vi "总磷通讯.vi"() -> ()   [LabVIEW 2016, in "斯坦道总磷.lvlib"]
uses:
  <vilib>/NI/Modbus Library/API/Wrapper/Create TCP Slave.vi
  <vilib>/Utility/config.llb/Write Key (Boolean).vi
  <vilib>/Utility/config.llb/Write Key (String).vi
  <vilib>/Plasmionique/MB Master/MB_Master/MB_Master.lvclass
  <vilib>/NI/Modbus Library/API/slave/Modbus Slave.lvclass
  <vilib>/Utility/config.llb/NI_LVConfig.lvlib
  <vilib>/Plasmionique/MB Master/MB Master.lvlib
  <vilib>/NI/Modbus Library/API/Wrapper/API Main.lvlib
panel:
  out "总氮测量数据区":u16[](array[numeric])
  out "总氮状态告警区":u16[](array[numeric])
  out "总磷状态告警区":u16[](array[numeric])
  out "总磷测量数据区":u16[](array[numeric])
  out "序列号":string
  out "状态告警区":T1
  out "测量数据区":T2 {"单位" items=["ug/L", "mg/L", "ppm", "mg/m3", "cm", "ppb", "ug/m3", "%", "nmol/mol", "umol/mol", "MPN/L", "MPN/100ml", "ng/m3", "NTU", "无量纲", "ms/cm", "us/cm", "℃", "mV", "万个/L"]}
  out "status":bool
  out "关键参数区":T3
  in  "读关键参数区":bool
  in  "读状态告警区":bool
  in  "读测量数据区":bool
  in  "站号":u16(ring) items=["总磷"=1, "氨氮"=3]
  in  "停止":bool
  in  "启动":bool
  in  "控制命令":u16(ring) items=["启动测量"=1, "标样核查"=2, "零点核查"=3, "跨度核查"=4, "空白测试"=5, "平行样测试"=6, "加标回收"=7, "空白校准"=8, "标样校准"=9, "初始化（清洗）"=10, "停止测试"=11, "仪器重启"=12, "校时"=13, "模式设置"=14, "测量间隔设置"=15]
  in  "控制命令参数":u16[](array[numeric]) format="%04xH"
  in  "VISA Resource":refnum<visa-resource-name>
  in  "启用模块":bool
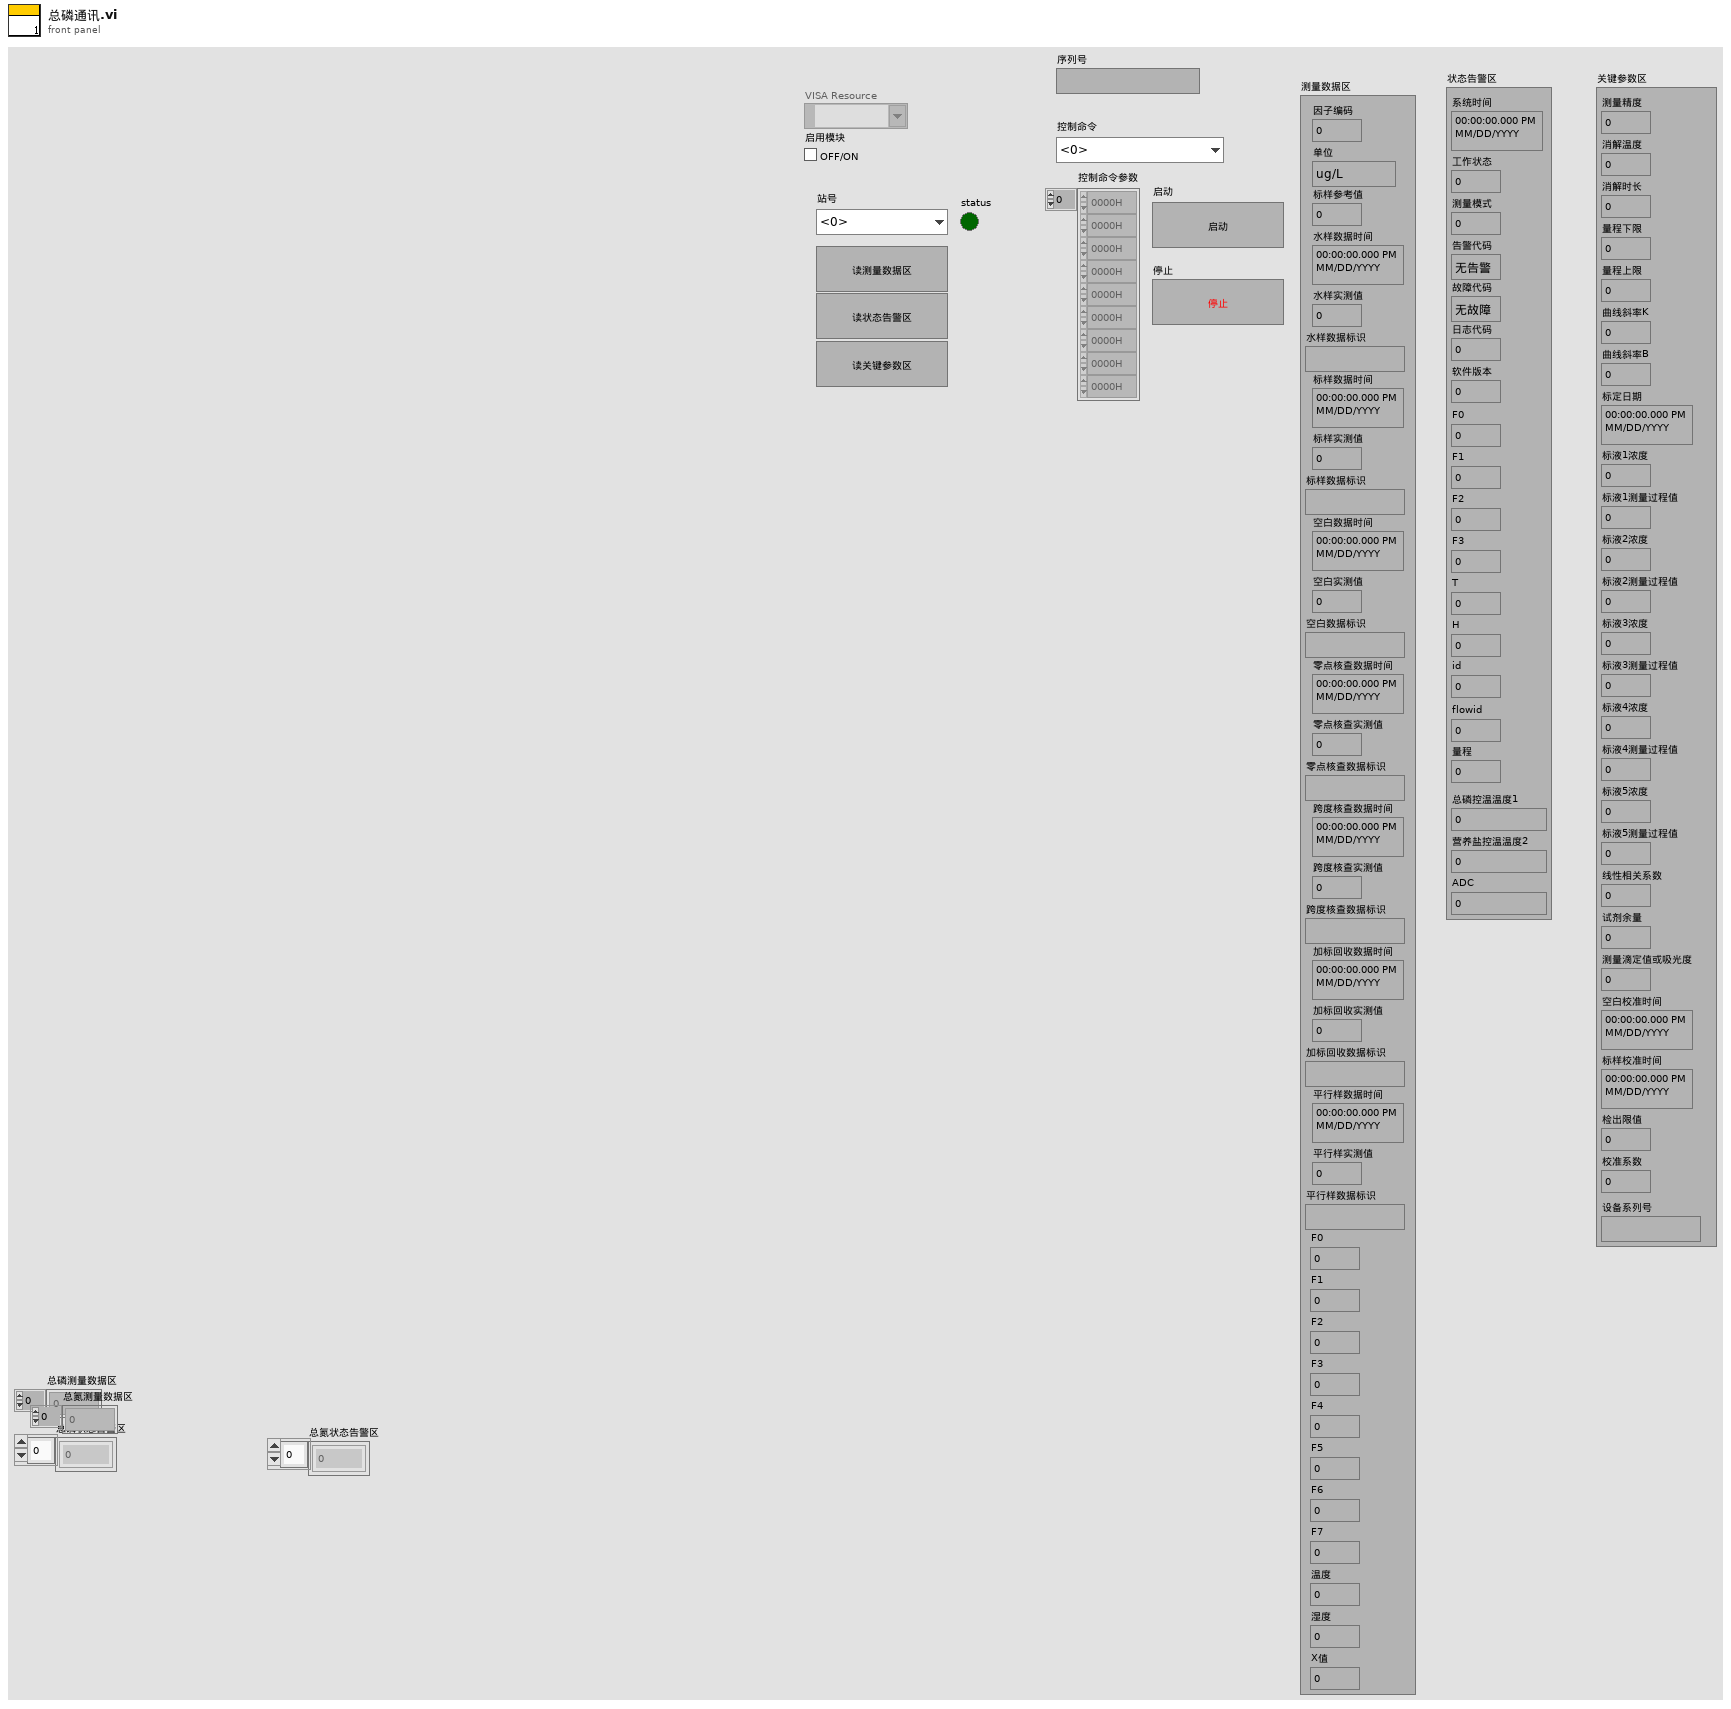
[diagram p1: front panel]
types:
  T1 = cluster{"系统时间":timestamp, "工作状态":u16, "测量模式":u16, "告警代码":enum16{"无告警", "缺试剂告警", "缺水样告警", "缺蒸馏水告警", "缺标液告警", "仪表漏液告警", "标定异常告警", "超量程告警", "加热异常", "低试剂预警", "超上限告警", "超下限告警", "仪表内部其他异常", "滴定异常告警", "电极异常告警", "量程切换告警", "参数设置告警", "PH电极电位异常", "电导率电极异常", "浊度光度异常", "溶解氧电极异常", "溶解氧光强异常", "温度异常告警", "PH异常告警", "溶解氧异常告警", "电导率异常告警", "浊度异常告警", "叶绿素异常告警", "藻密度异常告警", "蓝绿藻异常告警", "ORP异常告警", "氨氮异常告警", "清洁刷异常告警", "SD卡异常告警", "蓝牙异常告警", "Wifi异常告警", "流程异常告警"}, "故障代码":enum16{"无故障", "电机故障", "温度故障", "通讯故障", "滴定故障"}, "日志代码":u16, "软件版本":u16, "F0":sgl, "F1":sgl, "F2":sgl, "F3":sgl, "T":sgl, "H":sgl, "id":u16, "flowid":u16, "量程":u16, "总磷控温温度1":sgl, "营养盐控温温度2":sgl, "ADC":sgl}
  T2 = cluster{"因子编码":u32, "单位":u16, "标样参考值":sgl, "水样数据时间":timestamp, "水样实测值":sgl, "水样数据标识":string, "标样数据时间":timestamp, "标样实测值":sgl, "标样数据标识":string, "空白数据时间":timestamp, "空白实测值":sgl, "空白数据标识":string, "零点核查数据时间":timestamp, "零点核查实测值":sgl, "零点核查数据标识":string, "跨度核查数据时间":timestamp, "跨度核查实测值":sgl, "跨度核查数据标识":string, "加标回收数据时间":timestamp, "加标回收实测值":sgl, "加标回收数据标识":string, "平行样数据时间":timestamp, "平行样实测值":sgl, "平行样数据标识":string, "F0":sgl, "F1":sgl, "F2":sgl, "F3":sgl, "F4":sgl, "F5":sgl, "F6":sgl, "F7":sgl, "温度":sgl, "湿度":sgl, "X值":sgl}
  T3 = cluster{"测量精度":u16, "消解温度":u16, "消解时长":u16, "量程下限":sgl, "量程上限":sgl, "曲线斜率K":sgl, "曲线斜率B":sgl, "标定日期":timestamp, "标液1浓度":sgl, "标液1测量过程值":sgl, "标液2浓度":sgl, "标液2测量过程值":sgl, "标液3浓度":sgl, "标液3测量过程值":sgl, "标液4浓度":sgl, "标液4测量过程值":sgl, "标液5浓度":sgl, "标液5测量过程值":sgl, "线性相关系数":sgl, "试剂余量":u32, "测量滴定值或吸光度":sgl, "空白校准时间":timestamp, "标样校准时间":timestamp, "检出限值":sgl, "校准系数":sgl, "设备系列号":string}
  T4 = typedef "NI_LVConfig.lvlib/Config Data RefNum.ctl" = refnum<k1>
  T5 = enum8{"Enabled", "Disabled", "Disabled and Grayed Out"}
  T6 = cluster{"系统时间":timestamp, "工作状态":enum16{"空闲", "水样测试", "标样核查", "零点核查", "跨度核查", "空白测试", "平行样测试", "加标回收", "空白校准", "标样校准", "初始化（清洗）"}, "测量模式":enum16{"待机", "连续模式", "周期模式", "定点模式", "受控模式", "手动模式"}, "告警代码":enum16{"无告警", "缺试剂告警", "缺水样告警", "缺蒸馏水告警", "缺标液告警", "仪表漏液告警", "标定异常告警", "超量程告警", "加热异常", "低试剂预警", "超上限告警", "超下限告警", "仪表内部其他异常", "滴定异常告警", "电极异常告警", "量程切换告警", "参数设置告警", "PH电极电位异常", "电导率电极异常", "浊度光度异常", "溶解氧电极异常", "溶解氧光强异常", "温度异常告警", "PH异常告警", "溶解氧异常告警", "电导率异常告警", "浊度异常告警", "叶绿素异常告警", "藻密度异常告警", "蓝绿藻异常告警", "ORP异常告警", "氨氮异常告警", "清洁刷异常告警", "SD卡异常告警", "蓝牙异常告警", "Wifi异常告警", "流程异常告警"}, "故障代码":enum16{"无故障", "电机故障", "温度故障", "通讯故障", "滴定故障"}, "日志代码":u16, "软件版本":u16, "F0":sgl, "F1":sgl, "F2":sgl, "F3":sgl, "T":sgl, "H":sgl, "id":u16, "flowid":u16, "量程":u16, "总磷控温温度1":sgl, "营养盐控温温度2":sgl, "ADC":sgl}
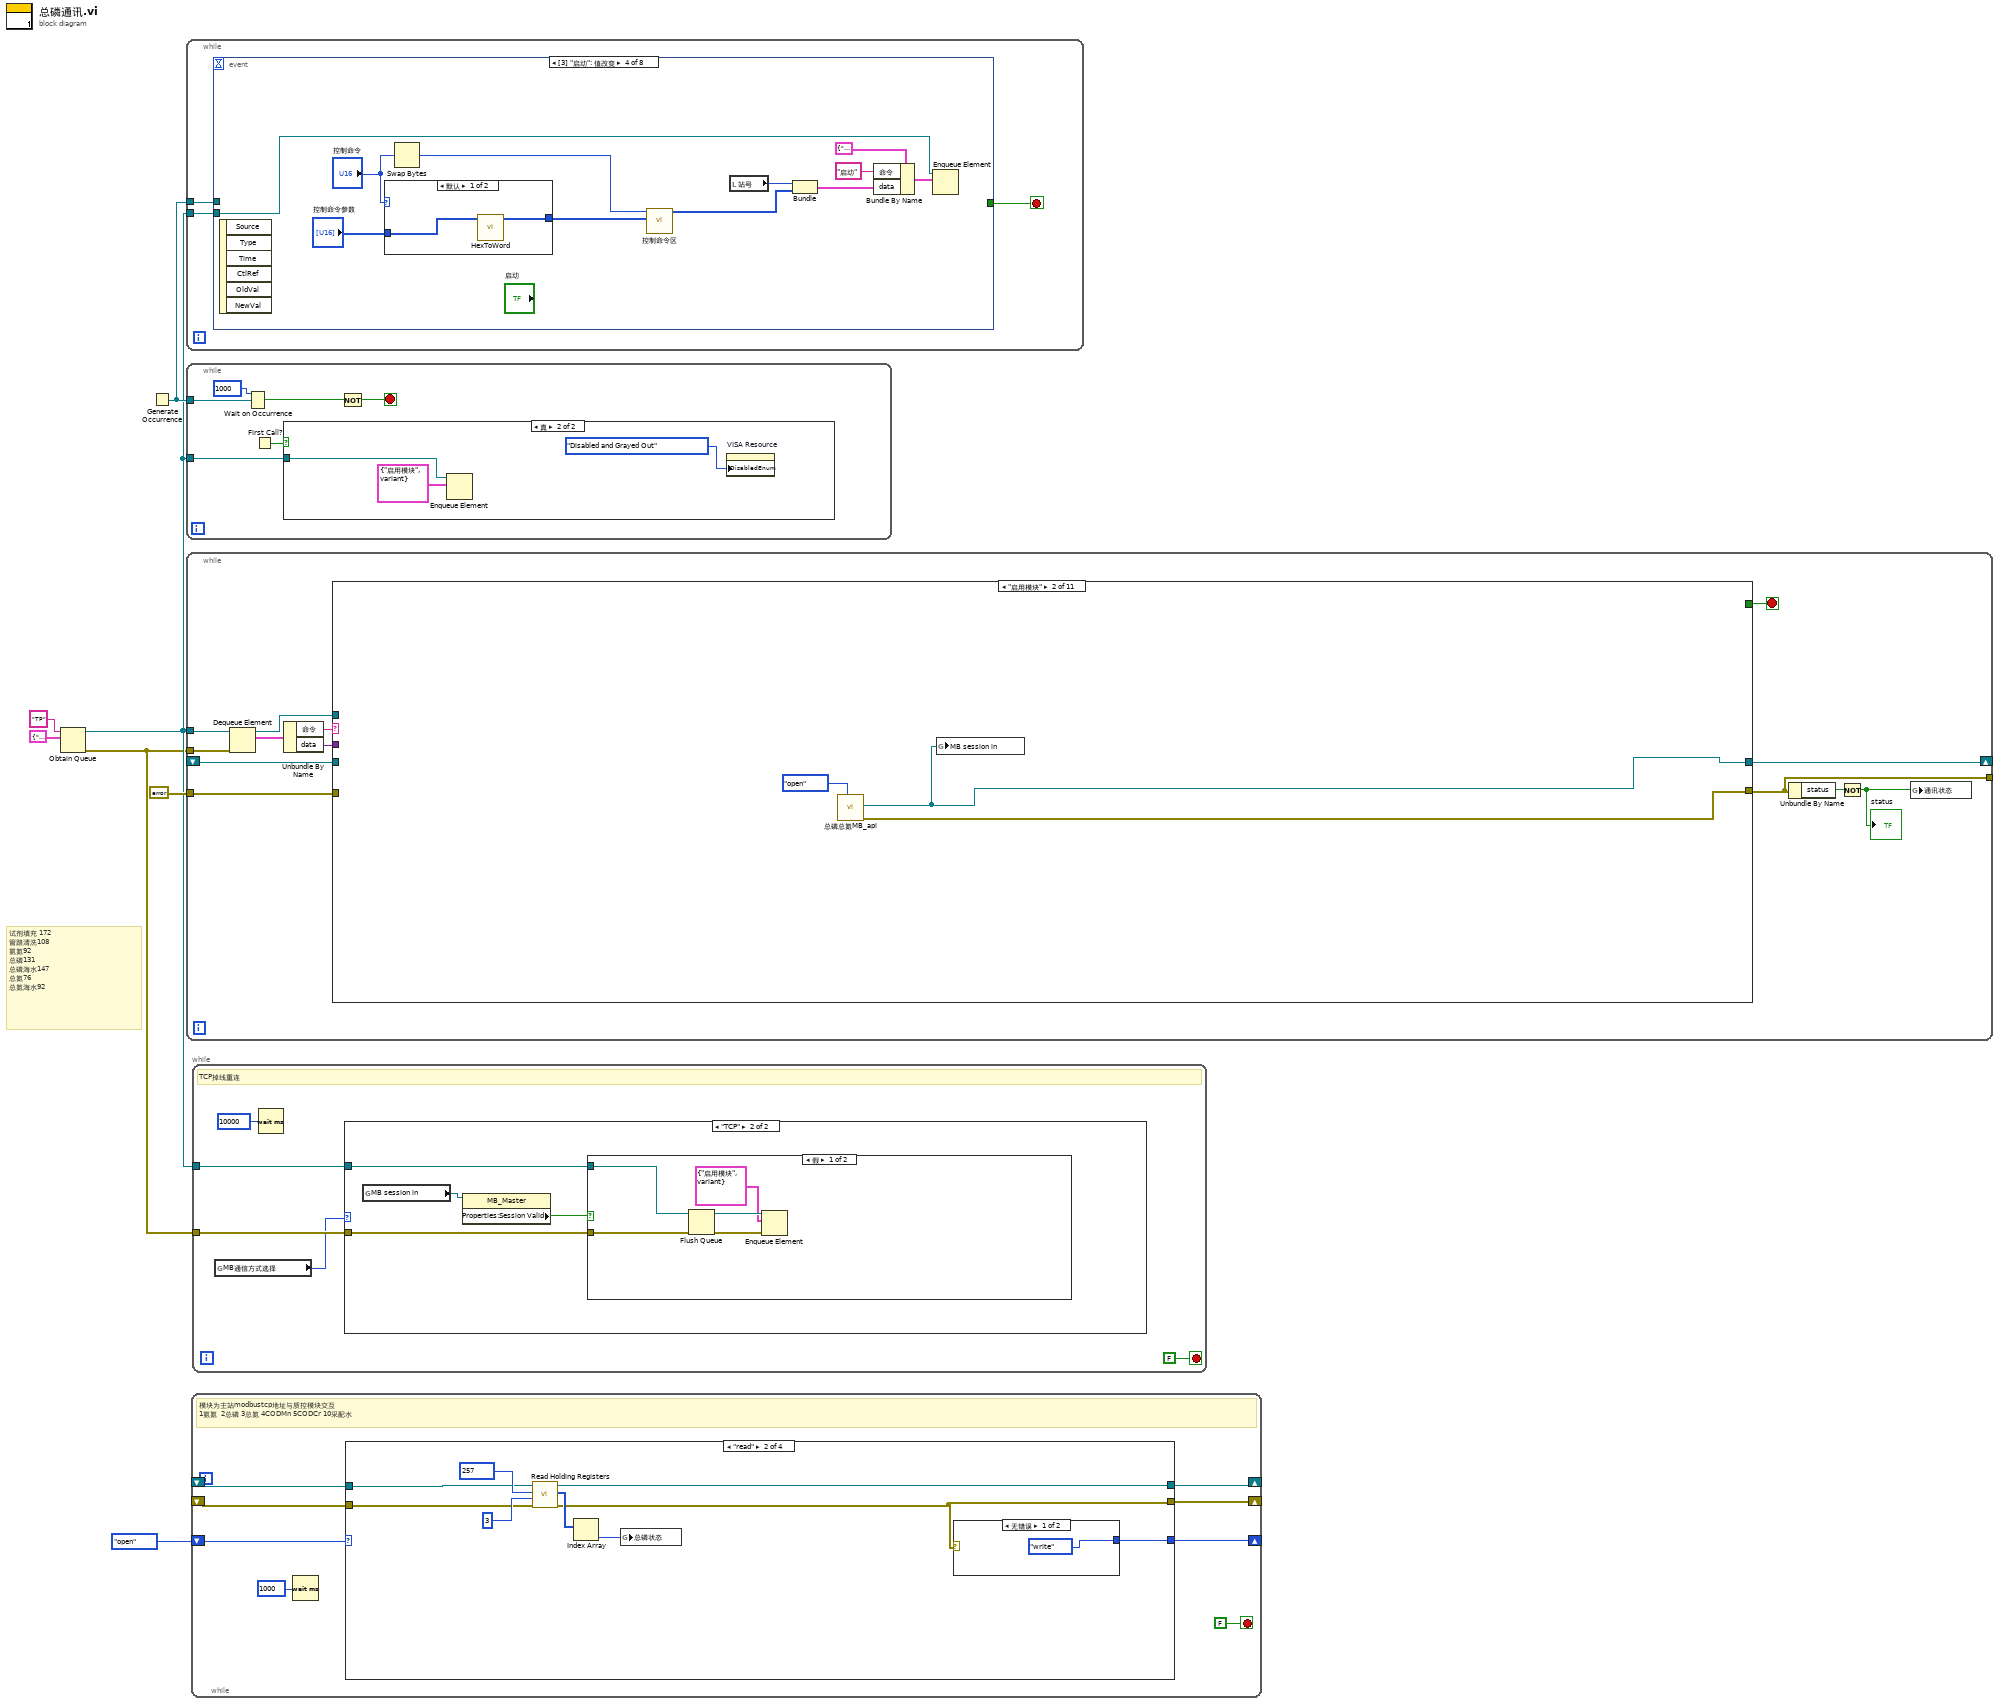
[diagram p0: block diagram]
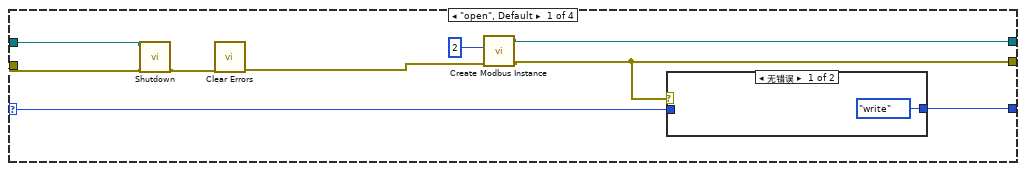
[diagram p4: hidden frame]
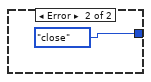
[diagram p6: hidden frame]
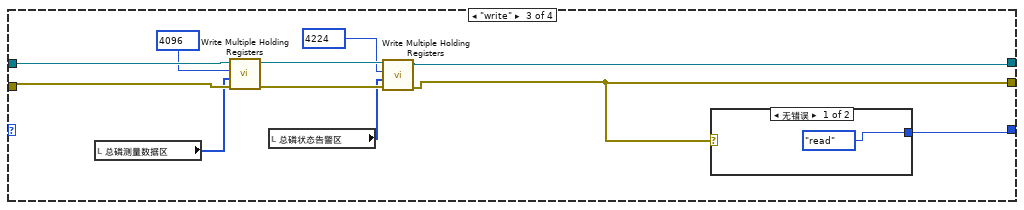
[diagram p7: hidden frame]
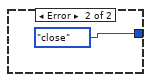
[diagram p8: hidden frame]
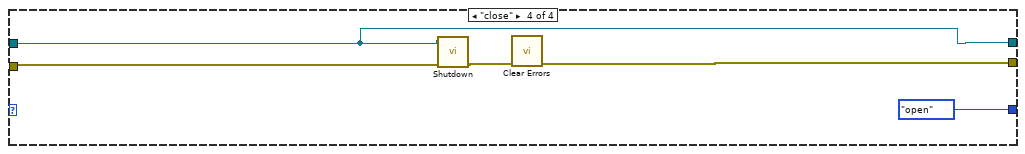
[diagram p9: hidden frame]
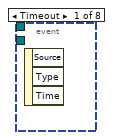
[diagram p11: hidden frame]
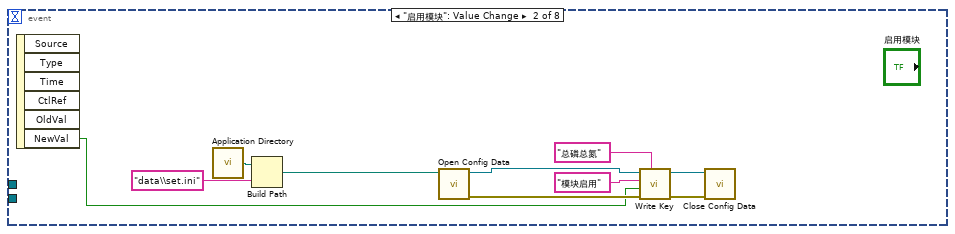
[diagram p12: hidden frame]
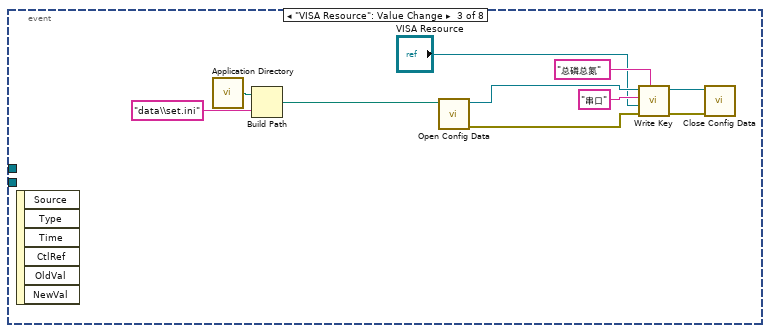
[diagram p13: hidden frame]
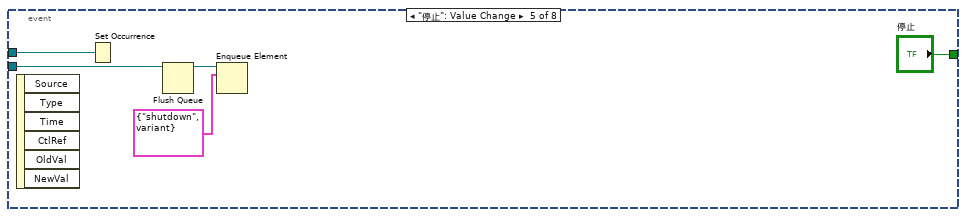
[diagram p15: hidden frame]
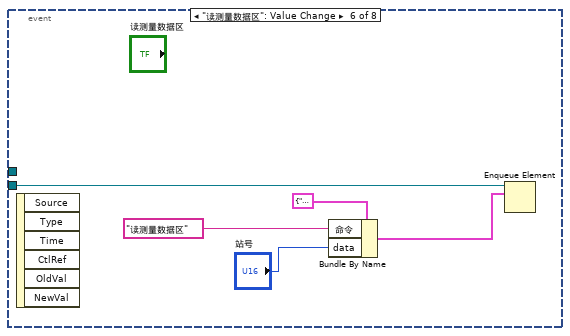
[diagram p16: hidden frame]
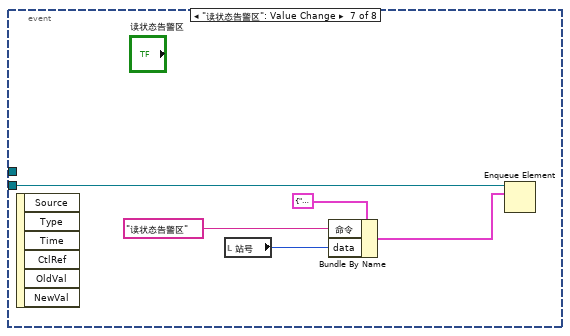
[diagram p17: hidden frame]
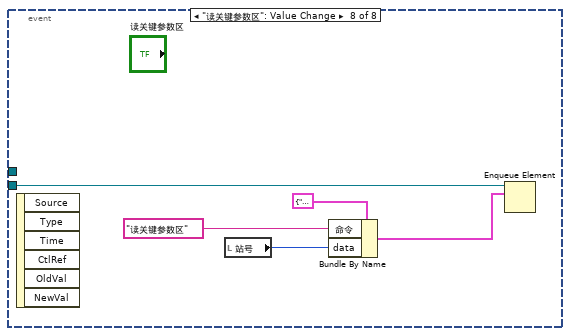
[diagram p18: hidden frame]
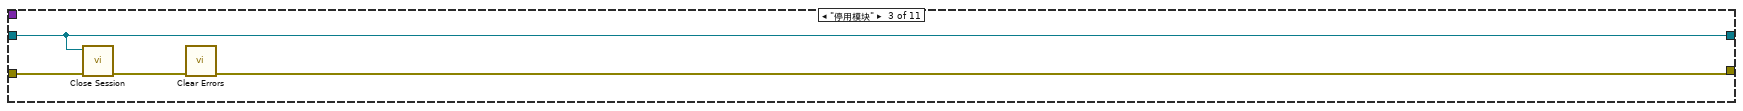
[diagram p20: hidden frame]
diagram:
  # "试剂填充 172 \n管路清洗108\n氨氮92\n总磷131\n总磷海水147\n总氮76\n总氮海水92"
  n1 = Obtain Queue(name (unnamed)="TP" ("名称（未命名）"), element data type=cluster{"命令":string, "data":variant} {"命令"="", "data"=variant}) -> (queue out=w2:refnum<queue>, error out=w1:errorcluster)  [unwired: 3 in, 1 out]
  n2 = Generate Occurrence() -> (w4:refnum<k4>)
  n3 = while {
    tunnel: w2 -> [w10]
    tunnel: w4 -> [w8]
    stop <- w9 stop-if-true
    n4 = event shown="[3] \"启动\": 值改变" {
      selector: _ -> [_ _ _ _ _ _ _ _]
      dyn-events: _ -> [_ _ _ _ _ _ _ _]
      timeout: _ -> [_ _ _ _ _ _ _ _]
      tunnel: w10 -> [_ _ _ w41 w48 w54 w59 w64]
      tunnel: [_ _ _ _ "停止" _ _ _] -> w9
      tunnel: w8 -> [_ _ _ _ w45 _ _ _]
      event Timeout {
        n5 = event-data() -> ()  [unwired: 1 in, 3 out]
      }
      event "启用模块": Value Change {
        n6 = event-data() -> ("NewVal"=w11:bool)  [unwired: 1 in, 5 out]
        n7 = call <vilib>:"Application Directory.vi"() -> ("Application Directory"=w13:path)
        n8 = Build Path(base path=w13, name or relative path="data\\set.ini" ("名称或相对路径")) -> (appended path=w14:path)
        n9 = call <vilib>:"Open Config Data.vi"("configuration file path"=w14) -> ("error out"=w20:errorcluster, "refnum"=w19:T4)  [unwired: 8 in, 1 out]
        n10 = call-poly <vilib>:"Write Key.vi"("section"="总磷总氮", "error in (no error)"=w20, "value"=w11, "key"="模块启用", "refnum"=w19) -> ("error out"=w16:errorcluster, "refnum out"=w12:T4)  [unwired: 4 in, 1 out]
        n11 = call <vilib>:"Close Config Data.vi"("error in (no error)"=w16, "refnum"=w12) -> ()  [unwired: 8 in, 2 out]
      }
      event "VISA Resource": Value Change {
        n12 = event-data() -> ()  [unwired: 1 in, 6 out]
        n13 = call <vilib>:"Application Directory.vi"() -> ("Application Directory"=w23:path)
        n14 = Build Path(base path=w23, name or relative path="data\\set.ini" ("名称或相对路径")) -> (appended path=w24:path)
        n15 = call <vilib>:"Open Config Data.vi"("configuration file path"=w24) -> ("error out"=w30:errorcluster, "refnum"=w29:T4)  [unwired: 8 in, 1 out]
        n16 = call-poly <vilib>:"Write Key.vi"("section"="总磷总氮", "error in (no error)"=w30, "value"="VISA Resource", "key"="串口", "refnum"=w29) -> ("error out"=w26:errorcluster, "refnum out"=w22:T4)  [unwired: 4 in, 1 out]
        n17 = call <vilib>:"Close Config Data.vi"("error in (no error)"=w26, "refnum"=w22) -> ()  [unwired: 8 in, 2 out]
      }
      event "启动": Value Change {
        n18 = event-data() -> ()  [unwired: 1 in, 6 out]
        n19 = case shown="默认" "控制命令" {
          tunnel: "控制命令参数" -> [w43 w44]
          tunnel: [w42 w44] -> w31
          frame Default {
            n20 = call "HexToWord.vi"("数组"=w43) -> ("WORD"=w42:u16[])  [unwired: 10 in]
          }
          frame 13 {
          }
        }
        n21 = Swap Bytes(anything="控制命令") -> (byte swapped=w34:u16)
        n22 = call "控制命令区.vi"("控制命令参数"=w31, "控制命令"=w34) -> ("控制命令"=w37:u16[])  [unwired: 9 in]
        n23 = local read "站号"() -> (w36:u16)
        n24 = Bundle("站号"=w36, "控制命令"=w37) -> (w35:cluster{"站号":u16, "控制命令":u16[]})  [unwired: 1 in]
        n25 = Bundle By Name(cluster=cluster{"命令":string, "data":variant} {"命令"="", "data"=variant} ("元素"), "命令"="启动", "data"=w35) -> (w39:cluster{"命令":string, "data":variant})
        n26 = Enqueue Element(queue=w41, element=w39) -> ()  [unwired: 2 in, 3 out]
      }
      event "停止": Value Change {
        n27 = event-data() -> ()  [unwired: 1 in, 6 out]
        n28 = Set Occurrence(w45) -> ()
        n29 = Flush Queue(queue=w48) -> (queue out=w47:refnum<queue>)  [unwired: 1 in, 2 out]
        n30 = Enqueue Element(queue=w47, element=cluster{"命令":string, "data":variant} {"命令"="shutdown", "data"=variant} ("元素")) -> ()  [unwired: 2 in, 3 out]
      }
      event "读测量数据区": Value Change {
        n31 = event-data() -> ()  [unwired: 1 in, 6 out]
        n32 = Bundle By Name(cluster=cluster{"命令":string, "data":variant} {"命令"="", "data"=variant} ("元素"), "命令"="读测量数据区", "data"="站号") -> (w52:cluster{"命令":string, "data":variant})
        n33 = Enqueue Element(queue=w54, element=w52) -> ()  [unwired: 2 in, 3 out]
      }
      event "读状态告警区": Value Change {
        n34 = event-data() -> ()  [unwired: 1 in, 6 out]
        n35 = local read "站号"() -> (w55:u16)
        n36 = Bundle By Name(cluster=cluster{"命令":string, "data":variant} {"命令"="", "data"=variant} ("元素"), "命令"="读状态告警区", "data"=w55) -> (w57:cluster{"命令":string, "data":variant})
        n37 = Enqueue Element(queue=w59, element=w57) -> ()  [unwired: 2 in, 3 out]
      }
      event "读关键参数区": Value Change {
        n38 = event-data() -> ()  [unwired: 1 in, 6 out]
        n39 = local read "站号"() -> (w60:u16)
        n40 = Bundle By Name(cluster=cluster{"命令":string, "data":variant} {"命令"="", "data"=variant} ("元素"), "命令"="读关键参数区", "data"=w60) -> (w62:cluster{"命令":string, "data":variant})
        n41 = Enqueue Element(queue=w64, element=w62) -> ()  [unwired: 2 in, 3 out]
      }
    }
  }
  n42 = while {
    tunnel: w4 -> [w70]
    tunnel: w2 -> [w66]
    stop <- w67 stop-if-true
    n43 = Wait on Occurrence(2:w70, 3:1000 ("毫秒超时(-1)")) -> (0:w68:bool)  [unwired: 1 in]
    n44 = First Call?() -> (First Call?: T/F=w65:bool)
    n45 = case shown="真" w65 {
      tunnel: w66 -> [_ w72]
      frame False {
      }
      frame True {
        n46 = Enqueue Element(queue=w72, element=cluster{"命令":string, "data":variant} {"命令"="启用模块", "data"=variant} ("元素")) -> ()  [unwired: 2 in, 3 out]
        n47 = property on="VISA Resource" class="VISAName"("DisabledEnum"=T5."Disabled and Grayed Out" ("禁用")) -> ()  [unwired: 2 in, 2 out]
      }
    }
    n48 = Not(x=w68) -> (.not. x?=w67:bool)
  }
  n49 = while {
    tunnel: w2 -> [w86]
    tunnel: w1 -> [w85]
    shift-right: [w83] -> _
    shift-left: _ -> [w82]
    tunnel: errorcluster {"status"=FALSE, "code"=0, "source"=""} ("error out") -> [w81]
    tunnel: [w76] -> _
    stop <- w84 stop-if-true
    n50 = Dequeue Element(queue=w86, error in (no error)=w85) -> (queue out=w77:refnum<queue>, element=w79:cluster{"命令":string, "data":variant})  [unwired: 1 in, 2 out]
    n51 = Unbundle By Name(w79) -> ("命令"=w80:string, "data"=w78:variant)
    n52 = case shown="\"启用模块\"" w80 {
      tunnel: w78 -> [_ _ _ w105 w116 w133 w143 w157 w175 w189 _]
      tunnel: w77 -> [_ _ _ _ _ _ _ _ _ _ w202]
      tunnel: [_ _ _ _ _ _ _ _ _ _ TRUE] -> w84
      tunnel: [w87 w90 w92 w108 w119 w135 w147 w166 w182 w196 w198] -> w83
      tunnel: [w88 w89 w93 w107 w118 w134 w148 w156 w183 w197 w199] -> w76
      tunnel: w82 -> [w87 _ w92 w104 w115 w132 w142 w160 w178 w192 w198]
      tunnel: w81 -> [w88 _ w95 w101 w112 w129 w140 w161 w179 w193 w200]
      frame Default {
      }
      frame "启用模块" {
        n53 = call "总磷总氮MB_api.vi"("STEP"=enum16{"open", "read", "write", "close"}."open") -> ("error out"=w89:errorcluster, "MB session out"=w90:refnum<class "MB_Master.lvclass">)  [unwired: 8 in, 1 out]
        n54 = global write "VAR总磷全局变量.vi" "MB session in"(w90) -> ()
      }
      frame "停用模块" {
        n55 = call-dynamic "Close Session.vi"("error in (no error)"=w95, "MB session in"=w92) -> ("error out"=w94:errorcluster)  [unwired: 9 in]
        n56 = call <vilib>:"Clear Errors.vi"("error in (no error)"=w94) -> ("error out"=w93:errorcluster)  [unwired: 5 in, 1 out]
      }
      frame "启动" {
        n57 = Variant To Data(type=cluster{"站号":u16, "控制命令":u16[]} {"站号"=0, "控制命令"=[]} ("输出簇"), Variant=w105) -> (data=w99:cluster{"站号":u16, "控制命令":u16[]})  [unwired: 1 in, 1 out]
        n58 = Unbundle By Name(w99) -> ("站号"=w98:u16, "控制命令"=w96:u16[])
        n59 = property class="MB_Master"(reference=w104, error in=w101, "Properties:Slave ID"=w98) -> (reference out=w103:refnum<class "MB_Master.lvclass">, error out=w102:errorcluster)
        n60 = Index Array(array=w96) -> (element=w97:u16)  [unwired: 1 in]
        n61 = global write "VAR总磷全局变量.vi" "控制命令"(w97) -> ()
        n62 = call <vilib>:"Write Multiple Registers.vi"("error in (no error)"=w102, "values"=w96, "starting address"=u16 4608, "MB session in"=w103) -> ("error out"=w107:errorcluster, "MB session out"=w108:refnum<class "MB_Master.lvclass">)  [unwired: 6 in]
      }
      frame "盲样测试" {
        n63 = Variant To Data(type=0, Variant=w116) -> (data=w109:i32)  [unwired: 1 in, 1 out]
        n64 = case shown="默认" w109 {
          tunnel: [u16[] [] ("values") u16[] [33539, 0] ("values") u16[] [23555, 0] ("values")] -> w111
          frame Default {
          }
          frame 1 {
            # "总磷盲样测试命令"
          }
          frame 3 {
            # "氨氮盲样测试"
          }
        }
        n65 = property class="MB_Master"(reference=w115, error in=w112, "Properties:Slave ID"=w109) -> (reference out=w114:refnum<class "MB_Master.lvclass">, error out=w113:errorcluster)
        n66 = call <vilib>:"Write Multiple Registers.vi"("error in (no error)"=w113, "values"=w111, "starting address"=u16 24592, "MB session in"=w114) -> ("error out"=w118:errorcluster, "MB session out"=w119:refnum<class "MB_Master.lvclass">)  [unwired: 6 in]
      }
      frame "debug" {
        n67 = Variant To Data(type=cluster{"站号":u16, "控制命令":u16[]} {"站号"=0, "控制命令"=[]} ("输出簇"), Variant=w133) -> (data=w127:cluster{"站号":u16, "控制命令":u16[]})  [unwired: 1 in, 1 out]
        n68 = Unbundle By Name(w127) -> ("站号"=w126:u16, "控制命令"=w124:u16[])
        n69 = property class="MB_Master"(reference=w132, error in=w129, "Properties:Slave ID"=w126) -> (reference out=w131:refnum<class "MB_Master.lvclass">, error out=w130:errorcluster)
        n70 = Index Array(array=w124) -> (element=w125:u16)  [unwired: 1 in]
        n71 = global write "VAR总磷全局变量.vi" "控制命令"(w125) -> ()
        n72 = call <vilib>:"Write Multiple Registers.vi"("error in (no error)"=w130, "values"=w124, "starting address"=u16 24594, "MB session in"=w131) -> ("error out"=w134:errorcluster, "MB session out"=w135:refnum<class "MB_Master.lvclass">)  [unwired: 6 in]
      }
      frame "读测量数据区" {
        n73 = Variant To Data(type=u8 1 ("Slave ID"), Variant=w143) -> (data=w138:u8)  [unwired: 1 in, 1 out]
        n74 = property class="MB_Master"(reference=w142, error in=w140, "Properties:Slave ID"=w138) -> (reference out=w141:refnum<class "MB_Master.lvclass">, error out=w139:errorcluster)
        n75 = call <vilib>:"Read Holding Registers.vi"("error in (no error)"=w139, "quantity"=u16 104, "starting address"=u16 4096, "MB session in"=w141) -> ("error out"=w148:errorcluster, "Registers"=w137:u16[], "MB session out"=w147:refnum<class "MB_Master.lvclass">)  [unwired: 5 in]
        n76 = call "测量数据区.vi"("数组"=w137) -> ("测量数据区"=w136:T2)  [unwired: 10 in]
        "测量数据区" <- w136
        n77 = case shown="2" w138 {
          tunnel: w136 -> [_ w149 w151]
          tunnel: w137 -> [_ w150 w152]
          frame 0, Default {
          }
          frame 1 {
            n78 = global write "VAR总磷全局变量.vi" "总磷测量数据区"(w149) -> ()
            "总磷测量数据区" <- w150
          }
          frame 2 {
            n79 = global write "VAR总磷全局变量.vi" "总氮测量数据区"(w151) -> ()
            "总氮测量数据区" <- w152
          }
        }
        n80 = global write "VAR总磷全局变量.vi" "测量数据区"(w136) -> ()
      }
      frame "读状态告警区" {
        n81 = Variant To Data(type=u8 1 ("Slave ID"), Variant=w157) -> (data=w162:u8)  [unwired: 1 in, 1 out]
        n82 = property class="MB_Master"(reference=w160, error in=w161, "Properties:Slave ID"=w162) -> (reference out=w159:refnum<class "MB_Master.lvclass">, error out=w158:errorcluster)
        n83 = call <vilib>:"Read Holding Registers.vi"("error in (no error)"=w158, "quantity"=u16 29, "starting address"=u16 4224, "MB session in"=w159) -> ("error out"=w156:errorcluster, "Registers"=w153:u16[], "MB session out"=w166:refnum<class "MB_Master.lvclass">)  [unwired: 5 in]
        n84 = call "状态告警区.vi"("数组"=w153) -> ("状态告警区"=w154:T6)  [unwired: 10 in]
        "状态告警区" <- w154
        n85 = global write "VAR总磷全局变量.vi" "状态告警区"(w154) -> ()
        n86 = Unbundle By Name(w154) -> ("id"=w155:u16)
        n87 = case shown="2, 76" w155 {
          tunnel: w154 -> [_ w167 w169]
          tunnel: w153 -> [_ w168 w170]
          frame 0, Default {
          }
          frame 1, 131 {
            n88 = global write "VAR总磷全局变量.vi" "总磷状态告警区"(w167) -> ()
            "总磷状态告警区" <- w168
          }
          frame 2, 76 {
            n89 = global write "VAR总磷全局变量.vi" "总氮状态告警区"(w169) -> ()
            "总氮状态告警区" <- w170
          }
        }
      }
      frame "读关键参数区" {
        n90 = Variant To Data(type=u8 1 ("Slave ID"), Variant=w175) -> (data=w173:u8)  [unwired: 1 in, 1 out]
        n91 = property class="MB_Master"(reference=w178, error in=w179, "Properties:Slave ID"=w173) -> (reference out=w177:refnum<class "MB_Master.lvclass">, error out=w176:errorcluster)
        n92 = call <vilib>:"Read Holding Registers.vi"("error in (no error)"=w176, "quantity"=u16 19, "starting address"=u16 4256, "MB session in"=w177) -> ("error out"=w183:errorcluster, "Registers"=w172:u16[], "MB session out"=w182:refnum<class "MB_Master.lvclass">)  [unwired: 5 in]
        n93 = call "关键参数区.vi"("数组"=w172) -> ("关键参数区"=w171:T3)  [unwired: 10 in]
        "关键参数区" <- w171
        n94 = global write "VAR总磷全局变量.vi" "关键参数区"(w171) -> ()
      }
      frame "读序列号" {
        n95 = Variant To Data(type=u8 1 ("Slave ID"), Variant=w189) -> (data=w187:u8)  [unwired: 1 in, 1 out]
        n96 = property class="MB_Master"(reference=w192, error in=w193, "Properties:Slave ID"=w187) -> (reference out=w191:refnum<class "MB_Master.lvclass">, error out=w190:errorcluster)
        n97 = call <vilib>:"Read Holding Registers.vi"("error in (no error)"=w190, "quantity"=u16 6, "starting address"=u16 3, "MB session in"=w191) -> ("error out"=w197:errorcluster, "Registers"=w186:u16[], "MB session out"=w196:refnum<class "MB_Master.lvclass">)  [unwired: 5 in]
        n98 = call "HexToString.vi"("数组"=w186) -> ("STRING"=w185:string[])  [unwired: 10 in]
        n99 = Index Array(array=w185) -> (element=w184:string)  [unwired: 1 in]
        "序列号" <- w184
        n100 = global write "VAR总磷全局变量.vi" "序列号"(w184) -> ()
      }
      frame "shutdown" {
        n101 = call-dynamic "Close Session.vi"("error in (no error)"=w200, "MB session in"=w198) -> ("error out"=w199:errorcluster)  [unwired: 9 in]
        n102 = Flush Queue(queue=w202) -> (queue out=w201:refnum<queue>)  [unwired: 1 in, 2 out]
        n103 = Release Queue(queue=w201) -> ()  [unwired: 2 in, 3 out]
      }
    }
    n104 = Unbundle By Name(w76) -> ("status"=w75:bool)
    n105 = Not(x=w75) -> (.not. x?=w74:bool)
    "status" <- w74
    n106 = global write "VAR总磷全局变量.vi" "通讯状态"(w74) -> ()
  }
  n107 = while {
    shift-right: [w209] -> _
    shift-left: _ -> [w211]
    shift-right: [w208] -> _
    shift-left: _ -> [w210]
    shift-right: [w205] -> _
    shift-left: enum16{"open", "read", "write", "close"}."open" -> [w206]
    stop <- FALSE stop-if-true
    # "模块为主站modbustcp地址与质控模块交互\n1氨氮  2总磷 3总氮 4CODMn 5CODCr 10采配水"
    n108 = Wait (ms)(milliseconds to wait=u32 1000 ("等待时间（毫秒）")) -> ()  [unwired: 1 out]
    n109 = case shown="\"read\"" w206 {
      selector: w206 -> [w220 _ _ _]
      tunnel: w211 -> [w214 w227 w243 w249]
      tunnel: w210 -> [w213 w226 w242 w248]
      tunnel: [w217 w225 w238 w249] -> w209
      tunnel: [w216 w224 w237 w251] -> w208
      tunnel: [w219 w231 w244 enum16{"open", "read", "write", "close"}."open"] -> w205
      frame "open", Default {
        n110 = call-dynamic "Shutdown.vi"("error in"=w213, "Modbus slave in"=w214) -> ("error out"=w212:errorcluster)  [unwired: 9 in]
        n111 = call <vilib>:"Clear Errors.vi"("error in (no error)"=w212) -> ("error out"=w215:errorcluster)  [unwired: 5 in, 1 out]
        n112 = call-poly <vilib>:"Create Modbus Instance.vi"("error in"=w215, "port (502)"=u16 2) -> ("error out"=w216:errorcluster, "TCP slave instance"=w217:refnum<class "Modbus Slave.lvclass">)  [unwired: 8 in]
        n113 = case shown="无错误" w216 {
          tunnel: w220 -> [_ w222]
          tunnel: [enum16{"open", "read", "write", "close"}."write" w222] -> w219
          frame No Error {
          }
          frame Error {
          }
        }
      }
      frame "read" {
        n114 = call-dynamic <vilib>:"Read Holding Registers.vi"("error in"=w226, "number of inputs"=u16 3, "starting address"=u16 257, "Modbus slave in"=w227) -> ("error out"=w224:errorcluster, "register values"=w228:u16[], "Modbus slave out"=w225:refnum<class "Modbus Slave.lvclass">)  [unwired: 5 in]
        n115 = Index Array(array=w228) -> (element=w223:u16)  [unwired: 1 in]
        n116 = global write "VAR总磷全局变量.vi" "总磷状态"(w223) -> ()
        n117 = case shown="无错误" w224 {
          tunnel: [enum16{"open", "read", "write", "close"}."write" enum16{"open", "read", "write", "close"}."close"] -> w231
          frame No Error {
          }
          frame Error {
          }
        }
      }
      frame "write" {
        n118 = local read "总磷测量数据区"() -> (w236:u16[])
        n119 = call-dynamic "Write Multiple Holding Registers.vi"("error in"=w242, "registers to write"=w236, "starting address"=u16 4096, "Modbus slave in"=w243) -> ("error out"=w239:errorcluster, "Modbus slave out"=w240:refnum<class "Modbus Slave.lvclass">)  [unwired: 6 in]
        n120 = local read "总磷状态告警区"() -> (w234:u16[])
        n121 = call-dynamic "Write Multiple Holding Registers.vi"("error in"=w239, "registers to write"=w234, "starting address"=u16 4224, "Modbus slave in"=w240) -> ("error out"=w237:errorcluster, "Modbus slave out"=w238:refnum<class "Modbus Slave.lvclass">)  [unwired: 6 in]
        n122 = case shown="无错误" w237 {
          tunnel: [enum16{"open", "read", "write", "close"}."read" enum16{"open", "read", "write", "close"}."close"] -> w244
          frame No Error {
          }
          frame Error {
          }
        }
      }
      frame "close" {
        n123 = call-dynamic "Shutdown.vi"("error in"=w248, "Modbus slave in"=w249) -> ("error out"=w247:errorcluster)  [unwired: 9 in]
        n124 = call <vilib>:"Clear Errors.vi"("error in (no error)"=w247) -> ("error out"=w251:errorcluster)  [unwired: 5 in, 1 out]
      }
    }
  }
  n125 = while "While循环" {
    tunnel: w2 -> [w254]
    tunnel: w1 -> [w253]
    stop <- FALSE stop-if-true
    # "TCP掉线重连"
    n126 = global read "总磷断电保存全局变量.vi" "MB通信方式选择"() -> (w252:enum16{"串口", "TCP"})
    n127 = Wait (ms)(milliseconds to wait=u32 10000 ("等待时间（毫秒）")) -> ()  [unwired: 1 out]
    n128 = case shown="\"TCP\"" w252 {
      tunnel: w254 -> [_ w259]
      tunnel: w253 -> [_ w258]
      frame "串口", Default {
      }
      frame "TCP" {
        n129 = global read "VAR总磷全局变量.vi" "MB session in"() -> (w257:refnum<class "MB_Master.lvclass">)
        n130 = property class="MB_Master"(reference=w257) -> ("Properties:Session Valid"=w260:bool)  [unwired: 1 in, 2 out]
        n131 = case shown="假" w260 {
          tunnel: w259 -> [w263 _]
          tunnel: w258 -> [w262 _]
          frame False {
            n132 = Flush Queue(queue=w263, error in (no error)=w262) -> (queue out=w265:refnum<queue>, error out=w264:errorcluster)  [unwired: 1 out]
            n133 = Enqueue Element(queue=w265, element=cluster{"命令":string, "data":variant} {"命令"="启用模块", "data"=variant} ("元素"), error in (no error)=w264) -> ()  [unwired: 1 in, 3 out]
          }
          frame True {
          }
        }
      }
    }
  }
